vi "SubVI-Template.vi"(8 "Err-I":errorcluster) -> (0 "Err-O":errorcluster)   [LabVIEW 2020]
doc: "CORE-ERROR HANDLING LOOP."
panel:
  # "Inputs"
  # "Outputs"
  # ":: SubVI with Error Handler ::\nby: HighTech <gaoke.yang@yahoo.com>\nhttp://www.mViAcademy.com\nCopyright (C) 2020, mVi Academy All Rights Reserved."
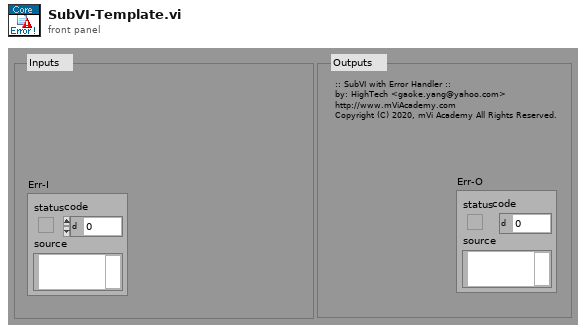
[diagram p1: front panel]
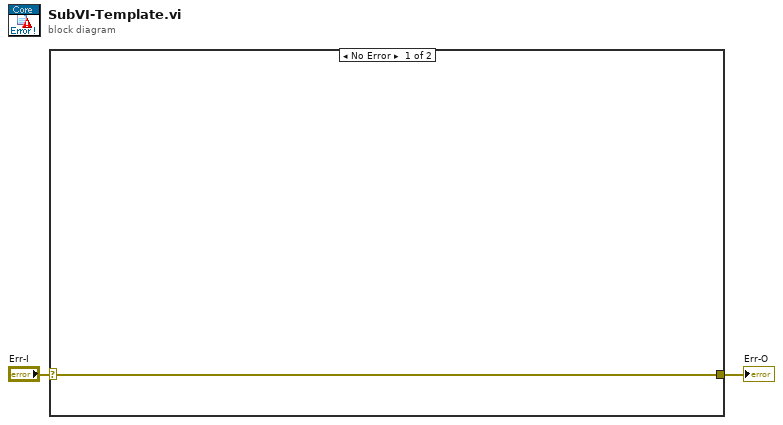
[diagram p0: block diagram]
diagram:
  n1 = case shown="No Error" "Err-I" {
    selector: "Err-I" -> [w3 w4]
    tunnel: [w3 w4] -> w1
    frame No Error {
    }
    frame Error {
    }
  }
  "Err-O" <- w1
